vi "Read Parent State.vi"(8 "error in (no error)":errorcluster, 11 "Nested State in":refnum<class "Nested State.lvclass">) -> (0 "error out":errorcluster, 2 "State.lvlib:State.lvclass":refnum<class "State.lvclass">, 3 "Nested State out":refnum<class "Nested State.lvclass">)   [LabVIEW 2024, in "Nested State.lvclass"]
uses:
  Nested State.lvclass
  State/State.lvclass
  Nested State.lvclass/Nested State.ctl
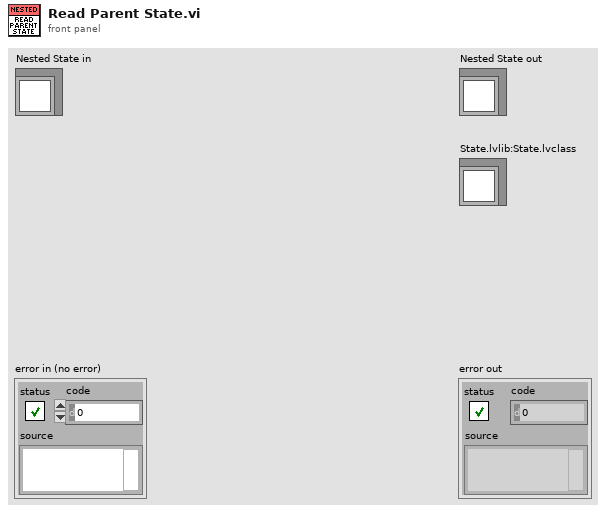
[diagram p1: front panel]
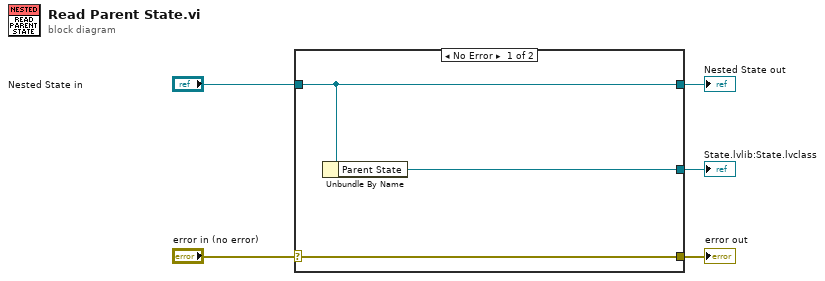
[diagram p0: block diagram]
diagram:
  n1 = case shown="No Error" "error in (no error)" {
    selector: "error in (no error)" -> [w8 w9]
    tunnel: [w8 w9] -> w4
    tunnel: [w7 w10] -> w2
    tunnel: "Nested State in" -> [w7 w10]
    tunnel: [w6 _] -> w1
    frame No Error {
      n2 = Unbundle By Name(w7) -> ("Parent State"=w6:refnum<class "State.lvclass">)
    }
    frame Error {
    }
  }
  "error out" <- w4
  "Nested State out" <- w2
  "State.lvlib:State.lvclass" <- w1
